vi "Error_Clear.vi"(8 "error in":errorcluster) -> (0 "error out (no error)":errorcluster)   [LabVIEW 2014, in "hse-misc.lvlib"]
doc: "Clears the error in <b>error in</b>\n\n\n\n____\nHAMPEL SOFTWARE ENGINEERING v0.7.0 (2018-07-16 18:12)"
uses:
  hse-misc.lvlib
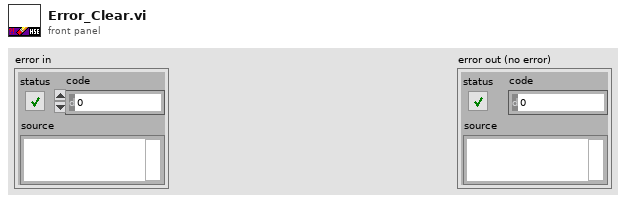
[diagram p1: front panel]
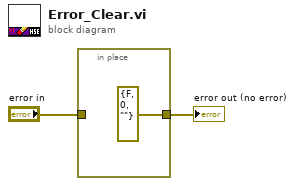
[diagram p0: block diagram]
diagram:
  n1 = in-place {
    in-place-border: [errorcluster {"status"=FALSE, "code"=0, "source"=""} ("error out")] -> w2
    in-place-border: "error in" -> [_]
  }
  "error out (no error)" <- w2
